vi "Get SubpanelVI Info.vi"(8 "error in (no error)":errorcluster, 11 "Hardware.lvlib:CCD.lvlib:CCD Configuration.lvclass":refnum<class "CCD Configuration.lvclass">) -> (0 "error out":errorcluster, 1 "Subpanel VI data":T1, 2 "Category string":string, 3 "reference out":refnum<class "CCD Configuration.lvclass">)   [LabVIEW 2016, in "Hardware.lvlib" / "CCD monitor.lvlib" / "CCD monitor configuration.lvclass"]
uses:
  <userlib>/Common Components/Hardware/Abstract System/Monitor/CCD monitor configuration.lvclass
  <userlib>/Configuration Dialog Actor/Methods/Data Retrieved by Lookup Table.ctl
  <userlib>/Configuration Dialog Actor/Configuration.lvclass
  <userlib>/Common Components/Hardware/CCD/CCD Configuration.lvclass
  <userlib>/Common Components/Hardware/CCD/CCD Configuration.lvclass/CCD Configuration.ctl
  <userlib>/Common Components/Hardware/Abstract Hardware/Hardware.lvclass/Hardware.ctl
  <userlib>/Common Components/Hardware/CCD/CCD Configuration/Read Hardware.lvlib_CCD.lvlib_CCD.lvclass.vi
  <userlib>/Common Components/Hardware/Abstract Hardware/Read Label.vi
  <userlib>/Common Components/Hardware/CCD/CCD/CCD.lvclass
  E:/NI LabVIEW/user.lib/Common Components/Hardware/Abstract Hardware/Hardware.lvclass
  <userlib>/Common Components/Hardware/CCD/CCD Configuration/Config CCD.vi
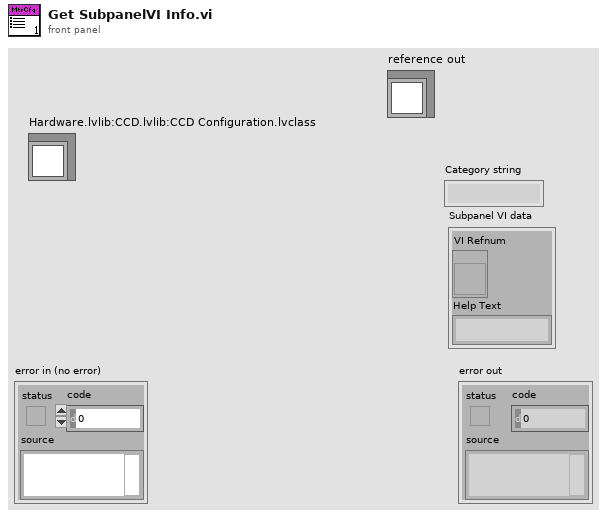
[diagram p1: front panel]
types:
  T1 = typedef "Configuration.lvlib/Configuration.lvclass/Data Retrieved by Lookup Table.ctl" = cluster{"VI Refnum":refnum<vi>, "Help Text":string}
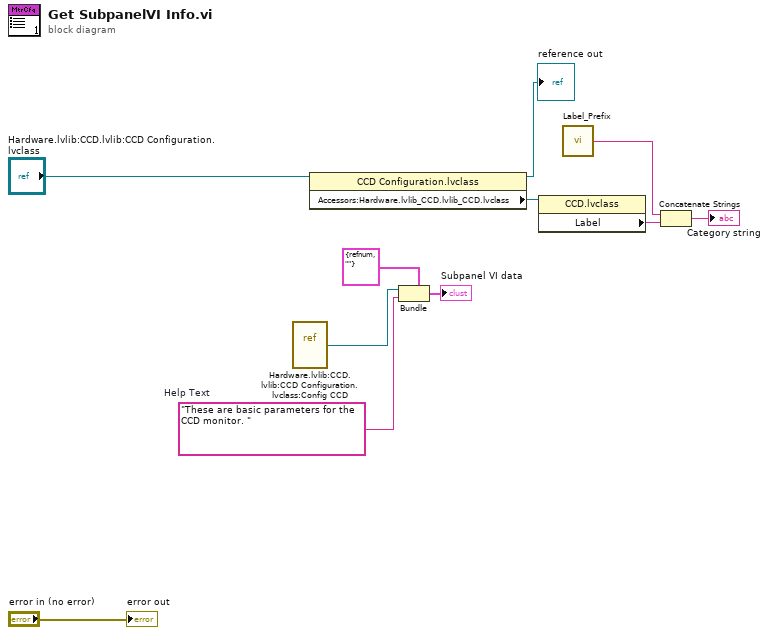
[diagram p0: block diagram]
diagram:
  w6 = "These are basic parameters for the CCD monitor. "  # Help Text
  n1 = vi-ref "Hardware.lvlib:CCD.lvlib:CCD Configuration.lvclass:Config CCD.vi"() -> (w7:refnum<vi>)
  n2 = property class="CCD Configuration.lvclass"(reference="Hardware.lvlib:CCD.lvlib:CCD Configuration.lvclass") -> (reference out=→"reference out":refnum<class "CCD Configuration.lvclass">, "Accessors:Hardware.lvlib_CCD.lvlib_CCD.lvclass"=w2:refnum<class "CCD.lvclass">)  [unwired: 1 in, 1 out]
  n3 = Bundle(cluster=T1 {"VI Refnum"=refnum, "Help Text"=""} ("output cluster"), "VI Refnum"=w7, "Help Text"=w6) -> (→"Subpanel VI data":T1)
  n4 = property class="CCD.lvclass"(reference=w2) -> ("Label"=w4:string)  [unwired: 1 in, 2 out]
  n5 = call <userlib>:"Label_Prefix.vi"() -> ("Label Prefix String"=w1:string)
  n6 = Concatenate Strings(w1, w4) -> (→"Category string":string)
  "error out" <- "error in (no error)"
